vi "DataDecoder.vi"(1 "byte":string="Ò") -> (0 "Data":i32)   [LabVIEW 2010]
doc: "Décodage d'un octet en valeur (8bits)"
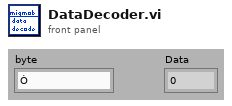
[diagram p1: front panel]
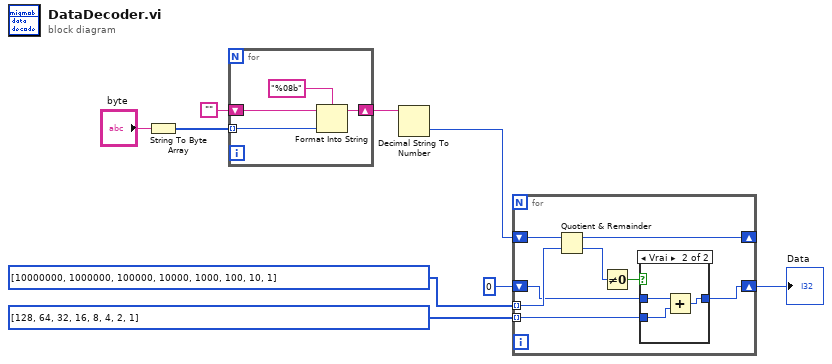
[diagram p0: block diagram]
diagram:
  n1 = String To Byte Array(string="byte") -> (unsigned byte array=w3:u8[])
  n2 = for {
    tunnel: w3 -> [w13] mode=indexing
    shift-right: [w11] -> w1
    shift-left: "" -> [w12]
    n3 = Format Into String(format string="%08b" ("chaîne de format"), initial string=w12, w13) -> (resulting string=w11:string)  [unwired: 1 in, 1 out]
  }
  n4 = Decimal String To Number(string=w1) -> (number=w7:i32)  [unwired: 2 in, 1 out]
  n5 = for {
    tunnel: i32[] [10000000, 1000000, 100000, 10000, 1000, 100, 10, 1] -> [w20] mode=indexing
    shift-right: [w16] -> _
    shift-left: w7 -> [w21]
    shift-right: [w14] -> w9
    shift-left: 0 -> [w17]
    tunnel: i32[] [128, 64, 32, 16, 8, 4, 2, 1] -> [w15] mode=indexing
    n6 = Quotient & Remainder(x=w21, y=w20) -> (x-y*floor(x/y)=w16:i32, floor(x/y)=w19:i32)
    n7 = Not Equal To 0?(x=w19) -> (x != 0?=w18:bool)
    n8 = case shown="Vrai" w18 {
      tunnel: w17 -> [w22 w25]
      tunnel: [w22 w23] -> w14
      tunnel: w15 -> [_ w24]
      frame False {
      }
      frame True {
        n9 = Add(x=w25, y=w24) -> (x+y=w23:i32)
      }
    }
  }
  "Data" <- w9
